vi "运行时序全局变量.vi"() -> ()   [LabVIEW 2016, in "斯坦道CODMn.lvlib"]
panel:
  out "多列列表框":i32(listbox)
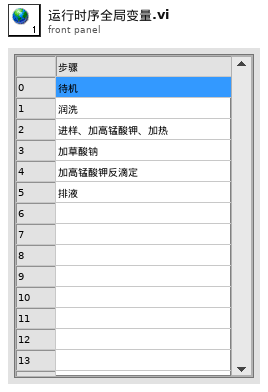
[diagram p1: front panel]
diagram:
